vi "Initialize Instrument.vi"(8 "error in (no error)":errorcluster, 10 "Reset":bool, 11 "Agilent 344xxA in":refnum<class "Agilent 344xxA.lvclass">) -> (0 "error out":errorcluster, 3 "Agilent 344xxA out":refnum<class "Agilent 344xxA.lvclass">)   [LabVIEW 2020, in "Agilent 344xxA.lvclass"]
uses:
  Agilent 344xxA.lvclass
  C:/Sandbox/Git_Sandbox/WiSpry Test Framework source code (LV20)/WiSpry Test Framework/Instruments/Instrument.lvclass
  Instrument.lvclass/Instrument.ctl
  Instrument.lvclass
  <instrlib>/Agilent 34401/Agilent 34401.lvlib
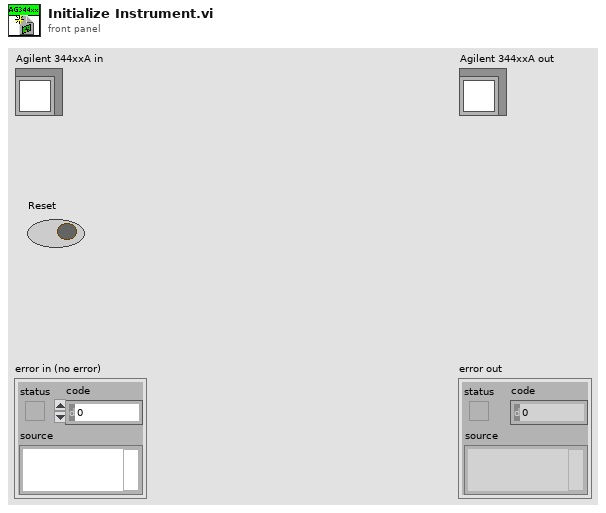
[diagram p1: front panel]
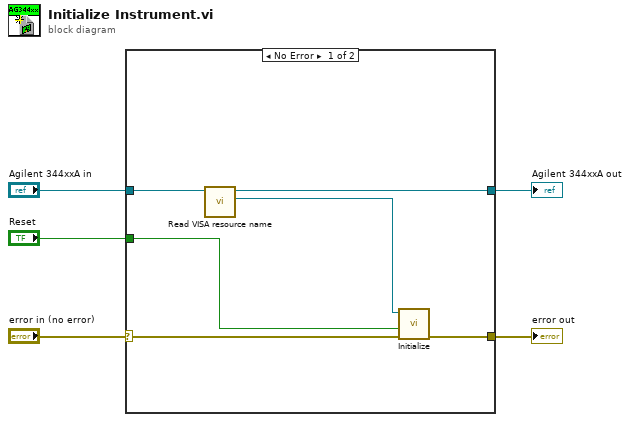
[diagram p0: block diagram]
diagram:
  n1 = case shown="No Error" "error in (no error)" {
    selector: "error in (no error)" -> [w10 w13]
    tunnel: [w6 w13] -> w4
    tunnel: "Agilent 344xxA in" -> [w11 w12]
    tunnel: [w7 w12] -> w2
    tunnel: "Reset" -> [w9 _]
    frame No Error {
      n2 = call "Read VISA resource name.vi"("Instrument in"=w11) -> ("VISA resource name"=w8:refnum<visa-resource-name>, "Instrument out"=w7:refnum<class "Agilent 344xxA.lvclass">)  [unwired: 9 in]
      n3 = call <instrlib>:"Initialize.vi"("error in (no error)"=w10, "Reset (True)"=w9, "VISA resource name"=w8) -> ("error out"=w6:errorcluster)  [unwired: 7 in, 1 out]
    }
    frame Error {
    }
  }
  "error out" <- w4
  "Agilent 344xxA out" <- w2
